vi "Calculate Injection Stage Times.vi"(7 "Sample rate (Hz)":u32, 11 "Injection Event Data Cluster":T1 {"Shot Info Array"."Results"."Off-Stage Avg Current" format="%#.6g"; "Shot Info Array"."Results"."Total Voltage Pulses" format="%#.6g"; "Shot Info Array"."Results"."Off-Stage Min Current" format="%#.6g"; "Shot Info Array"."Results"."Off-Stage Max Current" format="%#.6g"}) -> (3 "Injection Event Data Cluster out":T1 {"Shot Info Array"."Results"."Off-Stage Avg Current" format="%#.6g"; "Shot Info Array"."Results"."Total Voltage Pulses" format="%#.6g"; "Shot Info Array"."Results"."Off-Stage Min Current" format="%#.6g"; "Shot Info Array"."Results"."Off-Stage Max Current" format="%#.6g"})   [LabVIEW 2015, in "Fuel Injection Addon Engine.lvlib"]
uses:
  Fuel Injection Addon Engine.lvlib
  Types/Injector Event Data Cluster.ctl
  RT Analysis/Controls/Shot Information Control.ctl
  Types/Boost Stage Current Measurements Cluster Control.ctl
  Types/Async Parameters.ctl
  Shared/Types/Injector info.ctl
  <vilib>/NI Veristand/Custom Device API/Waveform Data Reference.ctl
  <vilib>/NI VeriStand/Custom Device Waveform API/Single Waveform Write (DBL)/Single Waveform Write (DBL).lvclass
  <vilib>/NI/NIVS Inline Async API/_Data Access Engine/Access Type Classes/Read/Read.lvclass
  <vilib>/NI/NIVS Inline Async API/_Data Access Engine/Access Type Classes/Write/Write.lvclass
  Shared/Types/Analysis.Channels.Select.ctl
  Shared/Constants.vi
  Shared/Fuel Injection Addon Shared.lvlib
  <vilib>/NI Veristand/Custom Device API/Custom Device API.lvlib
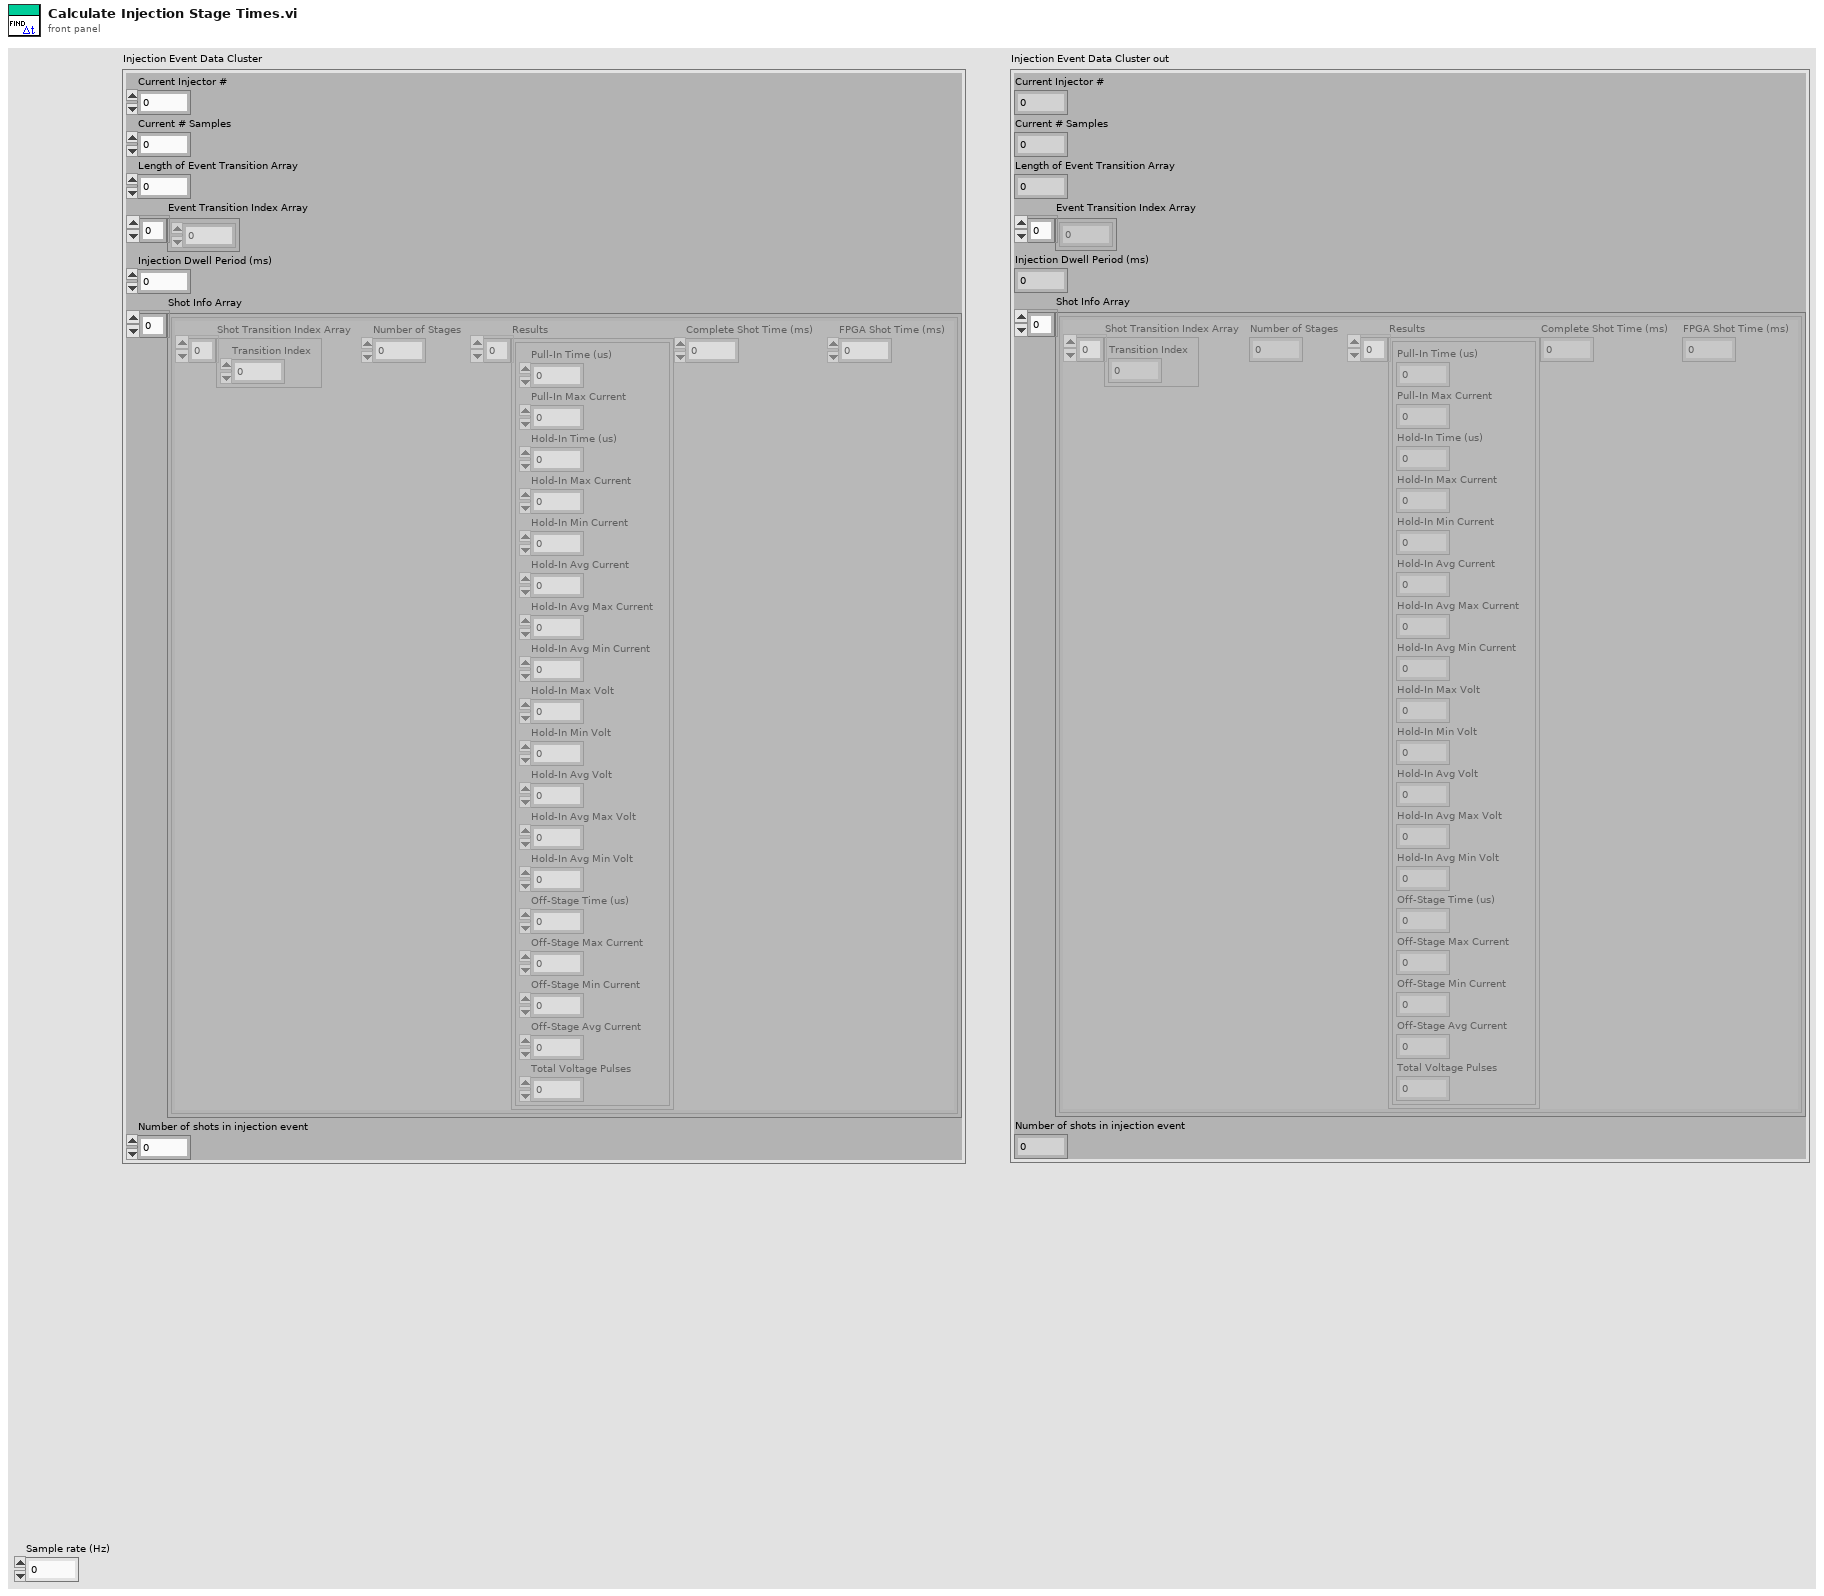
[diagram p1: front panel]
types:
  T1 = typedef "Fuel Injection Addon Engine.lvlib/Injector Event Data Cluster.ctl" = cluster{"Current Injector #":i16, "Current # Samples":i32, "Length of Event Transition Array":i16, "Event Transition Index Array":i32[], "Injection Dwell Period (ms)":dbl, "Shot Info Array":T2[], "Number of shots in injection event":i32}
  T2 = typedef "Fuel Injection Addon Engine.lvlib/Shot Information Control.ctl" = cluster{"Shot Transition Index Array":i32[], "Number of Stages":u16, "Results":T3[], "Complete Shot Time (ms) ":dbl, "FPGA Shot Time (ms)":dbl}
  T3 = typedef "Fuel Injection Addon Engine.lvlib/Boost Stage Current Measurements Cluster Control.ctl" = cluster{"Pull-In Time (us)":dbl, "Pull-In Max Current":dbl, "Hold-In Time (us)":dbl, "Hold-In Max Current":dbl, "Hold-In Min Current":dbl, "Hold-In Avg Current":dbl, "Hold-In Avg Max Current":dbl, "Hold-In Avg Min Current":dbl, "Hold-In Max Volt":dbl, "Hold-In Min Volt":dbl, "Hold-In Avg Volt":dbl, "Hold-In Avg Max Volt":dbl, "Hold-In Avg Min Volt":dbl, "Off-Stage Time (us)":dbl, "Off-Stage Max Current":dbl, "Off-Stage Min Current":dbl, "Off-Stage Avg Current":dbl, "Total Voltage Pulses":dbl}
  T4 = typedef "Fuel Injection Addon Engine.lvlib/Async Parameters.ctl" = cluster{"Name":string, "Sample rate (Hz)":u32, "Number of injectors":u8, "Max injection shot count":u8, "Injector info array":T5[], "Waveform data refs":T6[], "Waveform sessions refs":refnum<class "Single Waveform Write (DBL).lvclass">[], "DMA Ref":refnum<k20>, "WaveformEnable":refnum<data-value>, "Results":refnum<data-value>, "EventCounter":u64[], "FPGA Status":refnum<data-value>, "Analysis Selections":T7[], "Max Stages":u32, "Injector Timeout":dbl, "Timer":u32[], "Init Results Array":dbl[]}
  T5 = typedef "Fuel Injection Addon Shared.lvlib/Injector info.ctl" = cluster{"Results Index":i32, "Waveform Index":i32}
  T6 = typedef "Custom Device API.lvlib/Waveform Data Reference.ctl" = i32
  T7 = typedef "Fuel Injection Addon Shared.lvlib/Analysis.Channels.Select.ctl" = cluster{"Pull In Time":bool, "Pull In Max Current":bool, "Hold In Time":bool, "Hold In Max Current":bool, "Hold In Min Current":bool, "Hold In Avg Current":bool, "Hold In Avg Max Current":bool, "Hold In Avg Min Current":bool, "Hold In Max Volt":bool, "Hold In Min Volt":bool, "Hold In Avg Volt":bool, "Hold In Avg Max Volt":bool, "Hold In Avg Min Volt":bool, "Off Time":bool, "Off-Stage Max Current":bool, "Off-Stage Min Current":bool, "Off-Stage Avg Current":bool, "Total Voltage Pulses":bool}
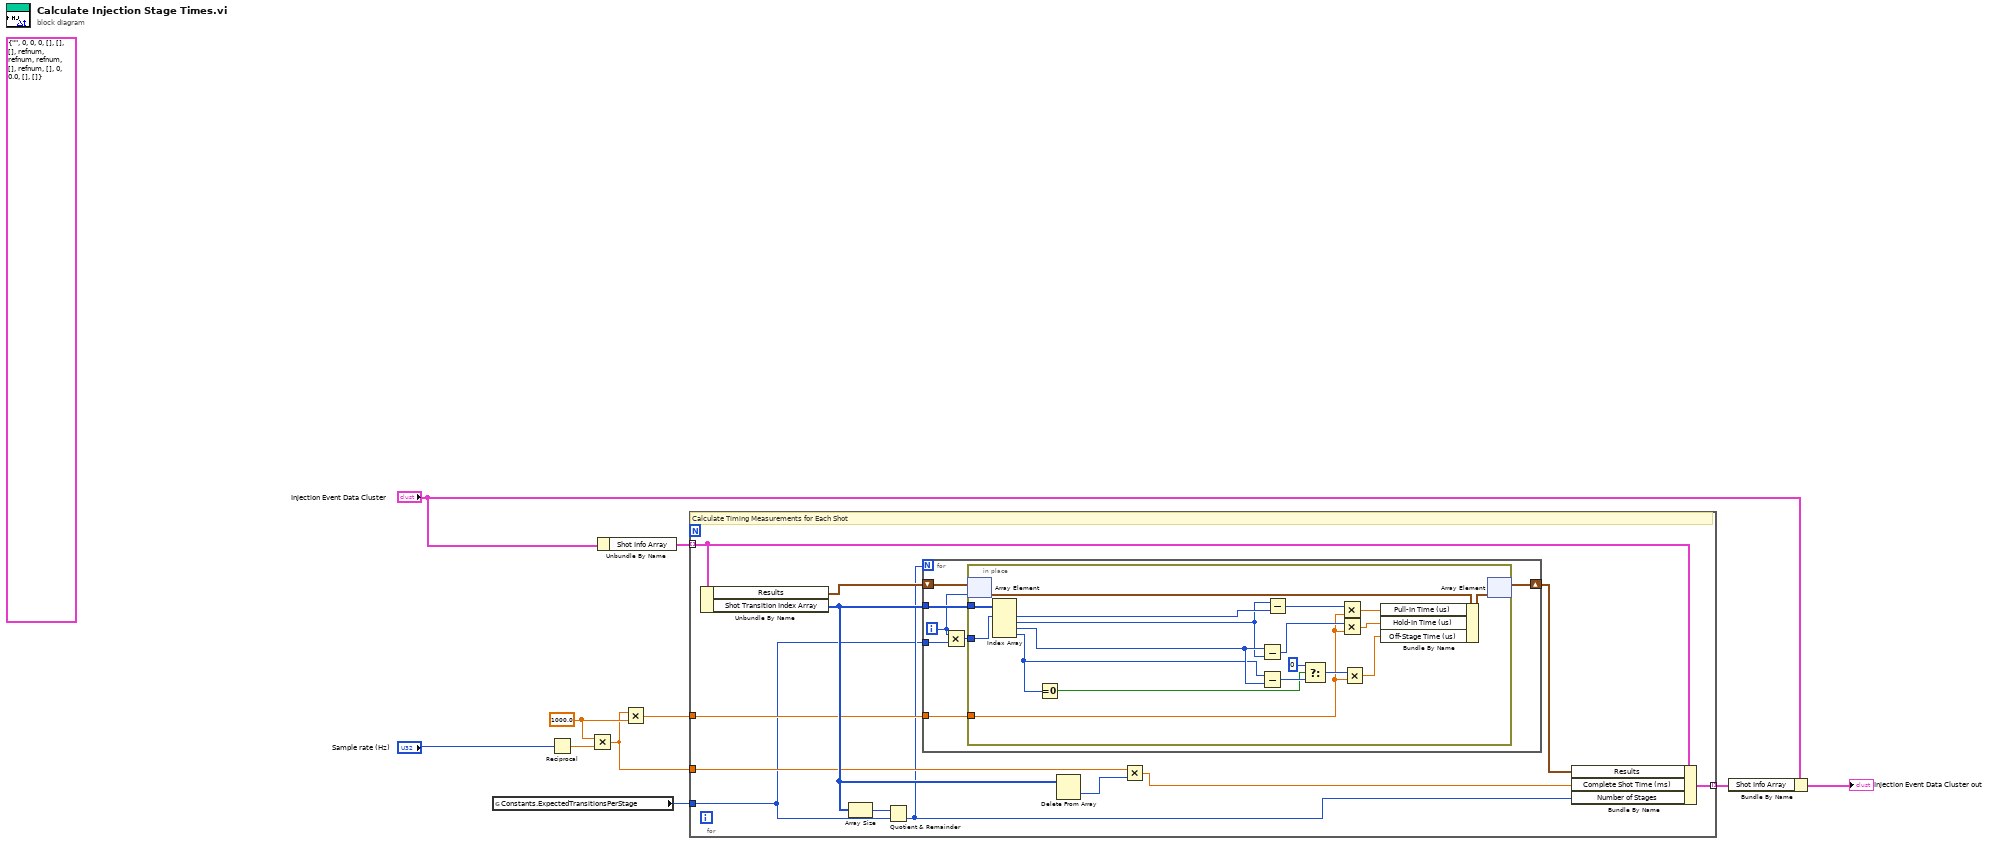
[diagram p0: block diagram]
diagram:
  w5 = 1000.0 ("y")
  (unwired) T4 {"Name"="", "Sample rate (Hz)"=0, "Number of injectors"=0, "Max injection shot count"=0, "Injector info array"=[], "Waveform data refs"=[], "Waveform sessions refs"=[], "DMA Ref"=refnum, "WaveformEnable"=refnum, "Results"=refnum, "EventCounter"=[], "FPGA Status"=refnum, "Analysis Selections"=[], "Max Stages"=0, "Injector Timeout"=0.0, "Timer"=[], "Init Results Array"=[]} ("Async Parameters")
  n1 = global read "Constants.vi" "Constants.ExpectedTransitionsPerStage"() -> (w2:u32)
  n2 = Reciprocal(x="Sample rate (Hz)") -> (1/x=w4:dbl)
  n3 = Multiply(x=w5, y=w4) -> (x*y=w1:dbl)
  n4 = Unbundle By Name("Injection Event Data Cluster") -> ("Shot Info Array"=w7:T2[])
  n5 = Multiply(x=w1, y=w5) -> (x*y=w3:dbl)
  n6 = for {
    tunnel: w7 -> [w22] mode=indexing
    tunnel: [w21] -> w6 mode=indexing
    tunnel: w1 -> [w16]
    tunnel: w3 -> [w13]
    tunnel: w2 -> [w11]
    # "Calculate Timing Measurements for Each Shot"
    n7 = Unbundle By Name(w22) -> ("Results"=w19:T3[], "Shot Transition Index Array"=w18:i32[])
    n8 = Array Size(array=w18) -> (size(s)=w20:i32)
    n9 = Quotient & Remainder(x=w20, y=w11) -> (floor(x/y)=w12:u32)  [unwired: 1 out]
    n10 = for {
      N: w12 -> [_]
      tunnel: w18 -> [w29]
      shift-right: [w25] -> w17
      shift-left: w19 -> [w28]
      tunnel: w13 -> [w24]
      tunnel: w11 -> [w23]
      i -> [w26]
      n11 = Multiply(x=w26, y=w23) -> (x*y=w27:u32)
      n12 = in-place {
        in-place-border: w29 -> [w46]
        in-place-border: w27 -> [w41]
        in-place-border: w24 -> [w30]
        n13 = in-place-array #1(w28, w26) -> (w43:T3)
        n14 = Index Array(array=w46, index #1=w41) -> (element #1=w45:i32, element #2=w44:i32, element #3=w47:i32, element #4=w40:i32)  [unwired: 3 in]
        n15 = Equal To 0?(x=w40) -> (x = 0?=w38:bool)
        n16 = Subtract(x=w47, y=w44) -> (x-y=w32:i32)
        n17 = Subtract(x=w40, y=w47) -> (x-y=w39:i32)
        n18 = Subtract(x=w44, y=w45) -> (x-y=w34:i32)
        n19 = Select(t=0, s=w38, f=w39) -> (s? t:f=w36:i32)
        n20 = Multiply(x=w34, y=w30) -> (x*y=w33:dbl)
        n21 = Multiply(x=w32, y=w30) -> (x*y=w31:dbl)
        n22 = Multiply(x=w36, y=w30) -> (x*y=w35:dbl)
        n23 = Bundle By Name(cluster=w43, "Pull-In Time (us)"=w33, "Hold-In Time (us)"=w31, "Off-Stage Time (us)"=w35) -> (w42:T3)
        n24 = in-place-array #1(w42) -> (w25:T3[])  [unwired: 1 out]
      }
    }
    n25 = Delete From Array(array=w18) -> (deleted portion=w15:i32)  [unwired: 2 in, 1 out]
    n26 = Multiply(x=w16, y=w15) -> (x*y=w14:dbl)
    n27 = Bundle By Name(cluster=w22, "Results"=w17, "Complete Shot Time (ms)"=w14, "Number of Stages"=w12) -> (w21:T2)
  }
  n28 = Bundle By Name(cluster="Injection Event Data Cluster", "Shot Info Array"=w6) -> (→"Injection Event Data Cluster out":T1)
